vi "command_delay.vi"(8 "error in (no error)":errorcluster, 10 "delay (ms) [deflaut = 5ms]":u32=5) -> (0 "error out":errorcluster)   [LabVIEW 2018]
doc: "A wait is needed after every command because the instrument cannot respond fast enough to subsequent commands immediately."
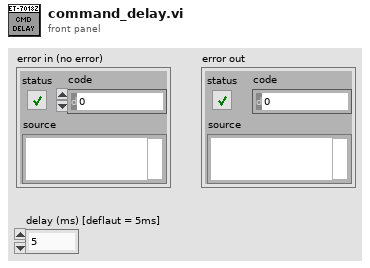
[diagram p1: front panel]
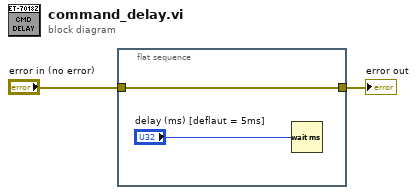
[diagram p0: block diagram]
diagram:
  n1 = flat-sequence {
    tunnel: "error in (no error)" -> [w4]
    tunnel: [w4] -> w2
    frame #0 {
      n2 = Wait (ms)(milliseconds to wait="delay (ms) [deflaut = 5ms]") -> ()  [unwired: 1 out]
    }
  }
  "error out" <- w2
